vi "Read socket.vi"(8 "error in (no error)":errorcluster, 11 "Detector in":refnum<class "Detector.lvclass">) -> (0 "error out":errorcluster, 2 "zeromq.lvlib:ZeroMQ Socket":refnum<class "zmq_socket.lvclass">, 3 "Detector out":refnum<class "Detector.lvclass">)   [LabVIEW 2018, in "Detector.lvclass"]
uses:
  Detector.lvclass
  <vilib>/addons/zeromq/zmq_socket.lvclass
  Detector.lvclass/Detector.ctl
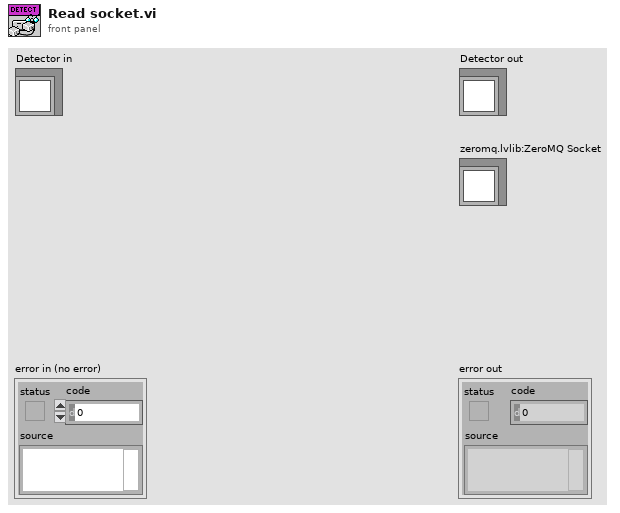
[diagram p1: front panel]
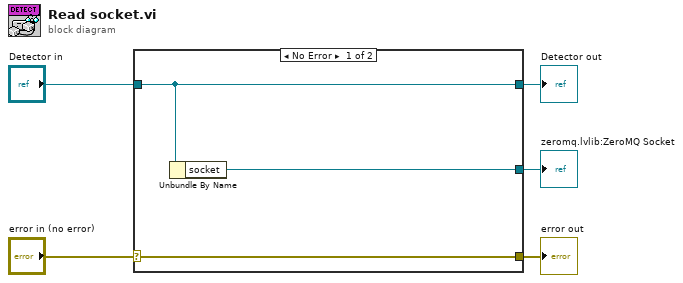
[diagram p0: block diagram]
diagram:
  n1 = case shown="No Error" "error in (no error)" {
    selector: "error in (no error)" -> [w8 w9]
    tunnel: [w8 w9] -> w4
    tunnel: [w7 w10] -> w2
    tunnel: "Detector in" -> [w7 w10]
    tunnel: [w6 _] -> w1
    frame No Error {
      n2 = Unbundle By Name(w7) -> ("socket"=w6:refnum<class "zmq_socket.lvclass">)
    }
    frame Error {
    }
  }
  "error out" <- w4
  "Detector out" <- w2
  "zeromq.lvlib:ZeroMQ Socket" <- w1
